vi "test.vi"() -> ()   [LabVIEW 2019]
uses:
  libtest.dll
panel:
  out "b 2":dbl
  out "a 2":dbl
  in  "b":dbl
  in  "a":dbl
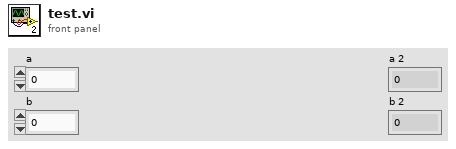
[diagram p1: front panel]
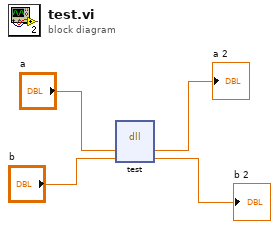
[diagram p0: block diagram]
diagram:
  n1 = dll-call lib="libtest.*" fn="test"("a"="a", "b"="b") -> ("a"=→"a 2":dbl, "b"=→"b 2":dbl)  [unwired: 4 in, 2 out]
